vi "Number to Letter.vi"(1 "Number":i32) -> (0 "Letter":string)   [LabVIEW 2019, in "SMO.Control Experiment.lvclass"]
uses:
  SMO.Control Experiment.lvclass
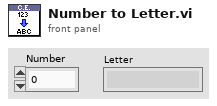
[diagram p1: front panel]
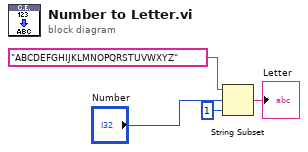
[diagram p0: block diagram]
diagram:
  n1 = String Subset(string="ABCDEFGHIJKLMNOPQRSTUVWXYZ", offset (0)="Number", length (rest)=1 ("length (rest)")) -> (substring=→"Letter":string)
